vi "Digital Input User Interface.vi"() -> ()   [LabVIEW 2023, in "GUI.lvlib" / "Diagnostic.lvlib"]
uses:
  Diagnostic.lvlib
  Control/Digital Input Cluster.ctl
  Control/Digital Input.ctl
  HardwareAbstractionLayer_LVOOP/Database/SQL Public VI/Control/DB Options.ctl
  HardwareAbstractionLayer_LVOOP/Main/Class Ref.ctl
  HardwareAbstractionLayer_LVOOP/DMM/DMM.lvclass
  HardwareAbstractionLayer_LVOOP/Function Generator/Function Generator.lvclass
  HardwareAbstractionLayer_LVOOP/Oscilloscope/Oscilloscope.lvclass
  HardwareAbstractionLayer_LVOOP/PowerSupply/PowerSupply.lvclass
  HardwareAbstractionLayer_LVOOP/Teststand/Teststand.lvclass
  HardwareAbstractionLayer_LVOOP/Analog Output/AO/AO.lvclass
  HardwareAbstractionLayer_LVOOP/Analog Input/AI/AI.lvclass
  HardwareAbstractionLayer_LVOOP/Database/Database.lvclass
  HardwareAbstractionLayer_LVOOP/Digital Output/DO_class/DO.lvclass
  HardwareAbstractionLayer_LVOOP/Digital Input/DI_class/DI.lvclass
  HardwareAbstractionLayer_LVOOP/PWM Output/PWM Output_class/PWM Output.lvclass
  HardwareAbstractionLayer_LVOOP/PWM Input/PWM Input_class/PWM Input.lvclass
  HardwareAbstractionLayer_LVOOP/NI Switch/NISwitch_class/NISwitch.lvclass
  HardwareAbstractionLayer_LVOOP/Modbus/Modbus_class/Modbus.lvclass
  HardwareAbstractionLayer_LVOOP/CAN/CAN Lib/CAN_class/CAN.lvclass
  HardwareAbstractionLayer_LVOOP/Digital Input/NI Digital Input_class/NI Digital Input.lvclass
  D:/eDCU LTT/VT LTT Project/Source Code/HardwareAbstractionLayer_LVOOP/Digital Input/DI_class/DI.lvclass
  HardwareAbstractionLayer_LVOOP/Main/Main.lvclass
  <userlib>/_OpenG.lib/appcontrol/appcontrol.llb/openg_application_control.lvlib
panel:
  in  "Stop Acquire":bool
  in  "Start Acquire":bool
  out "error out":errorcluster
  in  "error in":errorcluster
  in  "Operation":enum32{"6514-PXI2Slot9", "PXIe - SPARE"}(tab)
  out "PXIe - 6514_Digital Input":T1
  out "PXIe - 6514_Digital Input 2":T1
  in  "Stop":bool caption="Blank"
  # "Digital Input"
  # "Operation:"
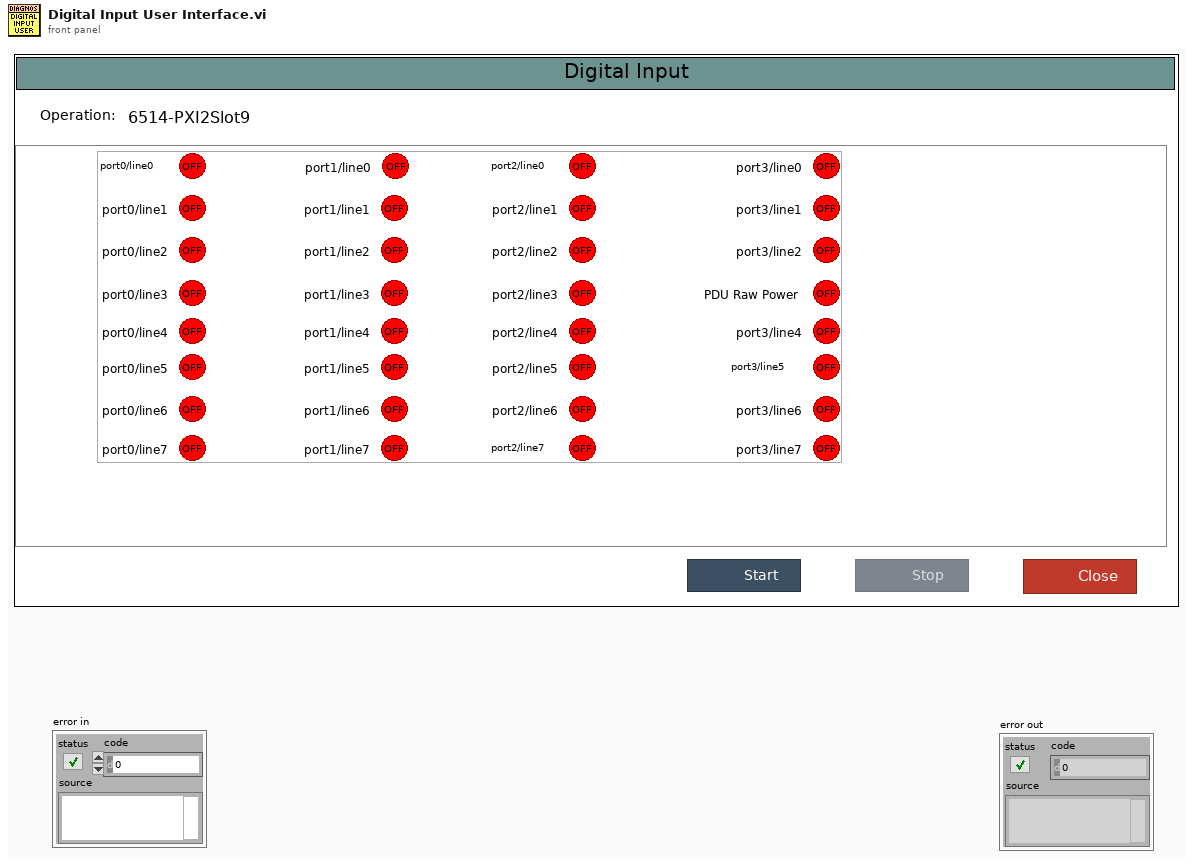
[diagram p1: front panel]
types:
  T1 = typedef "GUI.lvlib/Diagnostic.lvlib/Digital Input Cluster.ctl" = cluster{"Channel-0":T2, "Channel-1":T2, "Channel-2":T2, "Channel-3":T2, "Channel-4":T2, "Channel-5":T2, "Channel-6":T2, "Channel-7":T2, "Channel-8":T2, "Channel-9":T2, "Channel-10":T2, "Channel-11":T2, "Channel-12":T2, "Channel-13":T2, "Channel-14":T2, "Channel-15":T2, "Channel-16":T2, "Channel-17":T2, "Channel-18":T2, "Channel-19":T2, "Channel-20":T2, "Channel-21":T2, "Channel-22":T2, "Channel-23":T2, "Channel-24":T2, "Channel-25":T2, "Channel-26":T2, "Channel-27":T2, "Channel-28":T2, "Channel-29":T2, "Channel-30":T2, "Channel-31":T2}
  T2 = typedef "GUI.lvlib/Diagnostic.lvlib/Digital Input.ctl" = bool
  T3 = typedef "HardwareAbstractionLayer_LVOOP.lvlib/Database.lvclass/DB Options.ctl" = enum16{"Init", "Select Data", "Insert Data", "Update Data", "Delete Data", "Execute Query", "Create Schema", "Create Table", "List Tables", "List Columns", "Close"}
  T4 = typedef "HardwareAbstractionLayer_LVOOP.lvlib/Main.lvclass/Class Ref.ctl" = cluster{"DMM":refnum<class "DMM.lvclass">, "Function Generator":refnum<class "Function Generator.lvclass">, "Oscilloscope":refnum<class "Oscilloscope.lvclass">, "PowerSupply":refnum<class "PowerSupply.lvclass">, "Teststand":refnum<class "Teststand.lvclass">, "AO":refnum<class "AO.lvclass">, "AI":refnum<class "AI.lvclass">, "Database":refnum<class "Database.lvclass">, "AO Waveform Generation":refnum<class "AO.lvclass">, "DO":refnum<class "DO.lvclass">, "DI":refnum<class "DI.lvclass">, "PWM Output":refnum<class "PWM Output.lvclass">, "PWM Input":refnum<class "PWM Input.lvclass">, "RelayOutput":refnum<class "NISwitch.lvclass">, "Modbus":refnum<class "Modbus.lvclass">, "CAN":refnum<class "CAN.lvclass">}
  T5 = enum8{"Enabled", "Disabled", "Disabled and Grayed Out"}
  T6 = cluster{"data[0]":bool, "data[1]":bool, "data[2]":bool, "data[3]":bool, "data[4]":bool, "data[5]":bool, "data[6]":bool, "data[7]":bool, "data[8]":bool, "data[9]":bool, "data[10]":bool, "data[11]":bool, "data[12]":bool, "data[13]":bool, "data[14]":bool, "data[15]":bool, "data[16]":bool, "data[17]":bool, "data[18]":bool, "data[19]":bool, "data[20]":bool, "data[21]":bool, "data[22]":bool, "data[23]":bool, "data[24]":bool, "data[25]":bool, "data[26]":bool, "data[27]":bool, "data[28]":bool, "data[29]":bool, "data[30]":bool, "data[31]":bool}
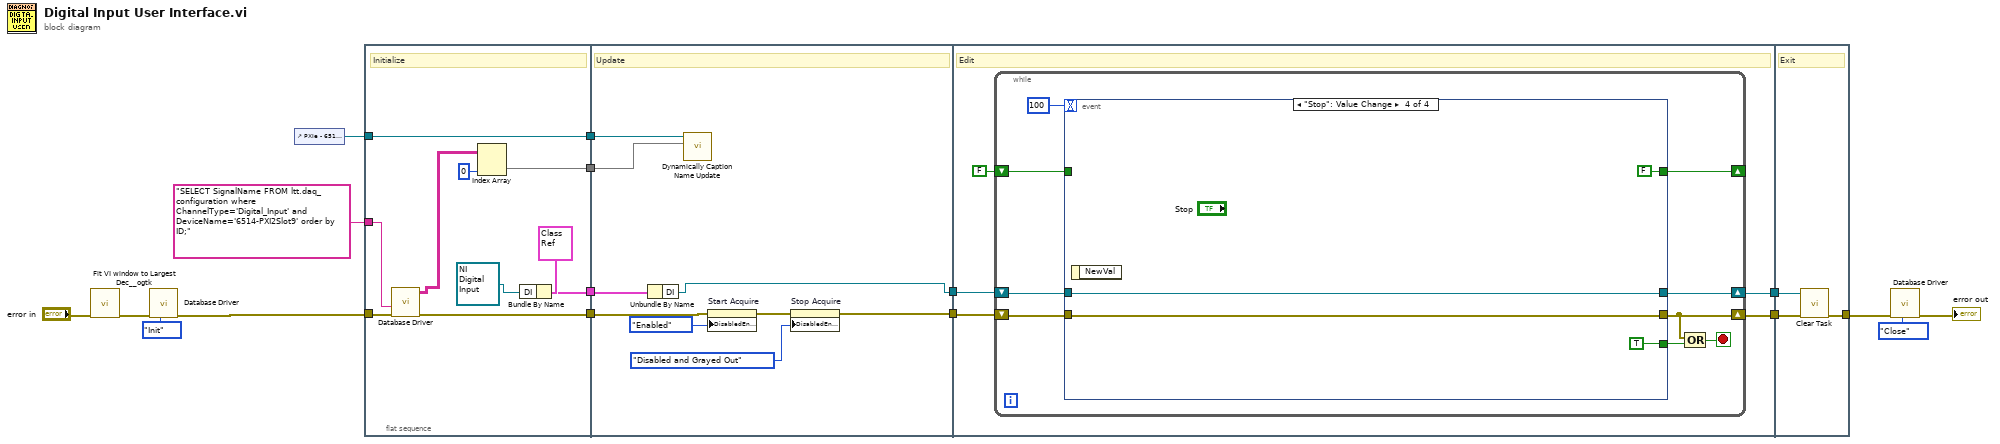
[diagram p0: block diagram]
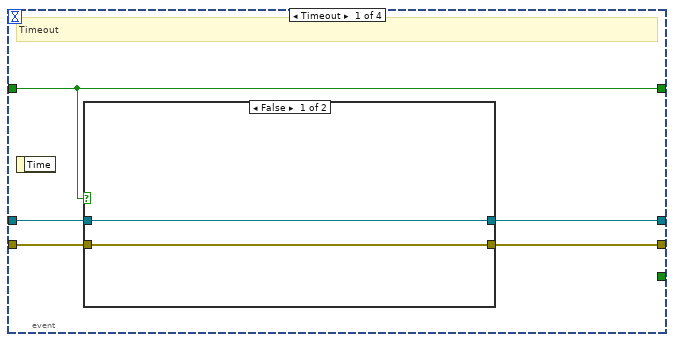
[diagram p2: hidden frame]
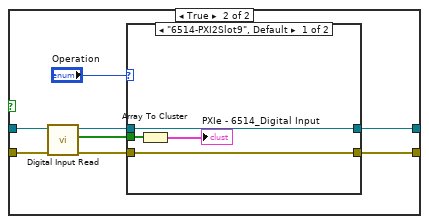
[diagram p3: hidden frame]
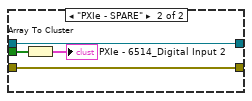
[diagram p4: hidden frame]
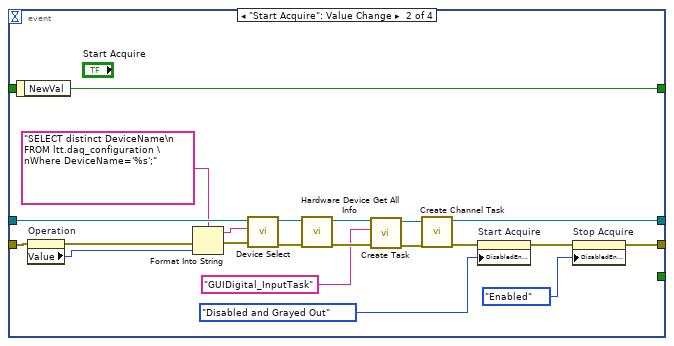
[diagram p5: hidden frame]
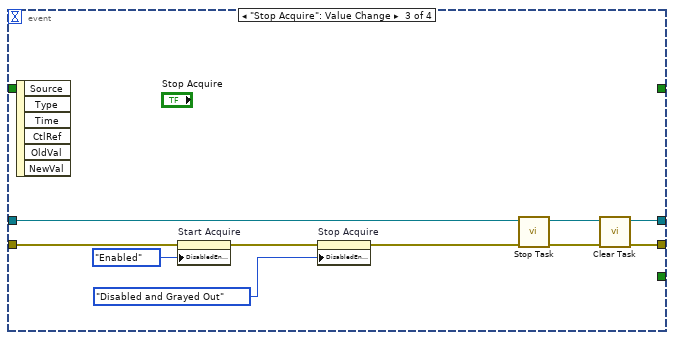
[diagram p6: hidden frame]
diagram:
  n1 = call <userlib>:"Fit VI window to Largest Dec__ogtk.vi"("error in (no error)"="error in") -> ("error out"=w1:errorcluster)  [unwired: 5 in, 1 out]
  n2 = call "Database Driver.vi"("Options"=DB_Options."Init", "error in"=w1) -> ("error out"=w11:errorcluster)  [unwired: 6 in, 3 out]
  n3 = control-ref of="PXIe - 6514_Digital Input"() -> (w5:refnum<vi>)
  n4 = flat-sequence {
    tunnel: [w21] -> w17
    tunnel: w11 -> [w22]
    tunnel: [w25] -> w16
    tunnel: w5 -> [w24]
    tunnel: [w24] -> w4
    tunnel: "SELECT SignalName FROM ltt.daq_configuration where ChannelType='Digital_Input' and DeviceName='6514-PXI2Slot9' order by ID;" -> [w23]
    tunnel: [w18] -> w2
    tunnel: w17 -> [w31]
    tunnel: w16 -> [w36]
    tunnel: [w35] -> w7
    tunnel: [w28] -> w6
    tunnel: w4 -> [w30]
    tunnel: w2 -> [w29]
    tunnel: [w41] -> w15
    tunnel: [w40] -> w14
    tunnel: w7 -> [w38]
    tunnel: w6 -> [w37]
    tunnel: [w111] -> w10
    tunnel: w15 -> [w109]
    tunnel: w14 -> [w110]
    frame #0 {
      # "Initialize"
      n5 = call "Database Driver.vi"("error in"=w22, "SQL query"=w23) -> ("error out"=w21:errorcluster, "data"=w20:string[][])  [unwired: 6 in, 2 out]
      n6 = Index Array(array=w20, index (col)=0 ("disabled index (col)")) -> (element=w18:string[])  [unwired: 1 in]
      n7 = Bundle By Name(cluster=T4 {"DMM"=refnum, "Function Generator"=refnum, "Oscilloscope"=refnum, "PowerSupply"=refnum, "Teststand"=refnum, "AO"=refnum, "AI"=refnum, "Database"=refnum, "AO Waveform Generation"=refnum, "DO"=refnum, "DI"=refnum, "PWM Output"=refnum, "PWM Input"=refnum, "RelayOutput"=refnum, "Modbus"=refnum, "CAN"=refnum} ("Class Cluster"), "DI"=refnum<class "NI Digital Input.lvclass"> refnum ("HardwareAbstractionLayer_LVOOP.lvlib:NI Digital Input.lvclass")) -> (w25:T4)
    }
    frame #1 {
      # "Update"
      n8 = Unbundle By Name(w36) -> ("DI"=w35:refnum<class "DI.lvclass">)
      n9 = call "Dynamically Caption Name Update.vi"("Caption Name"=w29, "Clust Refnum"=w30) -> ()  [unwired: 9 in, 1 out]
      n10 = property on="Start Acquire" class="Bool"(error in=w31, "DisabledEnum"=T5."Enabled" ("Disabled")) -> (error out=w34:errorcluster)  [unwired: 1 in, 1 out]
      n11 = property on="Stop Acquire" class="Bool"(error in=w34, "DisabledEnum"=T5."Disabled and Grayed Out" ("Disabled")) -> (error out=w28:errorcluster)  [unwired: 1 in, 1 out]
    }
    frame #2 {
      # "Edit"
      n12 = while {
        shift-right: [w45] -> w40
        shift-left: w38 -> [w47]
        shift-right: [w44] -> w41
        shift-left: w37 -> [w46]
        shift-right: [w43] -> _
        shift-left: FALSE ("NewVal") -> [w42]
        stop <- w48 stop-if-true
        n13 = event shown="[3] \"Stop\": Value Change" {
          selector: _ -> [_ _ _ _]
          dyn-events: _ -> [_ _ _ _]
          timeout: 100 -> [_ _ _ _]
          tunnel: [_ _ _ TRUE] -> w49
          tunnel: w47 -> [w52 w89 w95 w107]
          tunnel: w46 -> [w53 w84 w96 w106]
          tunnel: [w55 w74 w102 w106] -> w44
          tunnel: [w54 w85 w101 w107] -> w45
          tunnel: [w51 w94 _ FALSE ("NewVal")] -> w43
          tunnel: w42 -> [w51 _ _ _]
          event Timeout {
            # "Timeout"
            n14 = event-data() -> ()  [unwired: 1 in, 1 out]
            n15 = case shown="False" w51 {
              tunnel: [w56 w64] -> w55
              tunnel: [w57 w63] -> w54
              tunnel: w53 -> [w56 w62]
              tunnel: w52 -> [w57 w60]
              frame False {
              }
              frame True {
                n16 = call-dynamic "Digital Input Read.vi"("error in (no error)"=w62, "DI in"=w60) -> ("error out"=w61:errorcluster, "data"=w58:bool[], "DI out"=w59:refnum<class "DI.lvclass">)  [unwired: 7 in]
                n17 = case shown="\"6514-PXI2Slot9\", Default" "Operation" {
                  tunnel: w59 -> [w68 w73]
                  tunnel: w61 -> [w67 w72]
                  tunnel: [w67 w72] -> w64
                  tunnel: [w68 w73] -> w63
                  tunnel: w58 -> [w66 w70]
                  frame "6514-PXI2Slot9", Default {
                    n18 = Array To Cluster(array=w66) -> (cluster=→"PXIe - 6514_Digital Input":T6)
                  }
                  frame "PXIe - SPARE" {
                    n19 = Array To Cluster(array=w70) -> (cluster=→"PXIe - 6514_Digital Input 2":T6)
                  }
                }
              }
            }
          }
          event "Start Acquire": Value Change {
            n20 = event-data() -> ("NewVal"=w94:bool)  [unwired: 1 in]
            n21 = property on="Operation" class="TabCtl (strict)"(error in=w84) -> (error out=w83:errorcluster, "Value"=w80:enum32{"6514-PXI2Slot9", "PXIe - SPARE"})  [unwired: 1 in, 1 out]
            n22 = Format Into String(format string="SELECT distinct DeviceName\n FROM ltt.daq_configuration \nWhere DeviceName='%s';" ("SQL query"), error in=w83, w80) -> (resulting string=w82:string, error out=w79:errorcluster)  [unwired: 1 in]
            n23 = call-dynamic "Device Select.vi"("error in (no error)"=w79, "SQL query"=w82, "DI in"=w89) -> ("error out"=w92:errorcluster, "DI out"=w88:refnum<class "DI.lvclass">)  [unwired: 7 in]
            n24 = call-dynamic "Hardware Device Get All Info.vi"("error in (no error)"=w92, "DI in"=w88) -> ("error out"=w93:errorcluster, "DI out"=w87:refnum<class "DI.lvclass">)  [unwired: 8 in]
            n25 = call-dynamic "Create Task.vi"("error in (no error)"=w93, "Task name"="GUIDigital_InputTask", "DI in"=w87) -> ("error out"=w90:errorcluster, "DI out"=w86:refnum<class "DI.lvclass">)  [unwired: 7 in]
            n26 = call-dynamic "Create Channel Task.vi"("error in (no error)"=w90, "DI in"=w86) -> ("error out"=w75:errorcluster, "DI out"=w85:refnum<class "DI.lvclass">)  [unwired: 8 in]
            n27 = property on="Start Acquire" class="Bool"(error in=w75, "DisabledEnum"=T5."Disabled and Grayed Out" ("Disabled")) -> (error out=w78:errorcluster)  [unwired: 1 in, 1 out]
            n28 = property on="Stop Acquire" class="Bool"(error in=w78, "DisabledEnum"=T5."Enabled" ("Disabled")) -> (error out=w74:errorcluster)  [unwired: 1 in, 1 out]
          }
          event "Stop Acquire": Value Change {
            n29 = event-data() -> ()  [unwired: 1 in, 6 out]
            n30 = property on="Start Acquire" class="Bool"(error in=w96, "DisabledEnum"=T5."Enabled" ("Disabled")) -> (error out=w97:errorcluster)  [unwired: 1 in, 1 out]
            n31 = property on="Stop Acquire" class="Bool"(error in=w97, "DisabledEnum"=T5."Disabled and Grayed Out" ("Disabled")) -> (error out=w98:errorcluster)  [unwired: 1 in, 1 out]
            n32 = call-dynamic "Stop Task.vi"("error in (no error)"=w98, "DI in"=w95) -> ("error out"=w99:errorcluster, "DI out"=w100:refnum<class "DI.lvclass">)  [unwired: 8 in]
            n33 = call-dynamic "Clear Task.vi"("error in (no error)"=w99, "DI in"=w100) -> ("error out"=w102:errorcluster, "DI out"=w101:refnum<class "DI.lvclass">)  [unwired: 8 in]
          }
          event "Stop": Value Change {
            n34 = event-data() -> ()  [unwired: 1 in, 1 out]
          }
        }
        n35 = Compound Arithmetic op=OR(w44, w49) -> (w48:bool)
      }
    }
    frame #3 {
      # "Exit"
      n36 = call-dynamic "Clear Task.vi"("error in (no error)"=w109, "DI in"=w110) -> ("error out"=w111:errorcluster)  [unwired: 8 in, 1 out]
    }
  }
  n37 = call "Database Driver.vi"("Options"=DB_Options."Close", "error in"=w10) -> ("error out"=→"error out":errorcluster)  [unwired: 6 in, 3 out]
